vi "Tenney Calculate Setpoint Change.vi"(0 "Average":dbl, 1 "Adjustment Amount":dbl, 5 "Target Upper limit":dbl, 7 "Target Lower limit":dbl, 11 "error in (no error)":errorcluster, 12 "Chamber Upper limit":dbl, 13 "Chamber Lower limit":dbl, 14 "Chamber Setpoint":dbl) -> (4 "new_setpoint":dbl, 15 "error out":errorcluster)   [LabVIEW 2023]
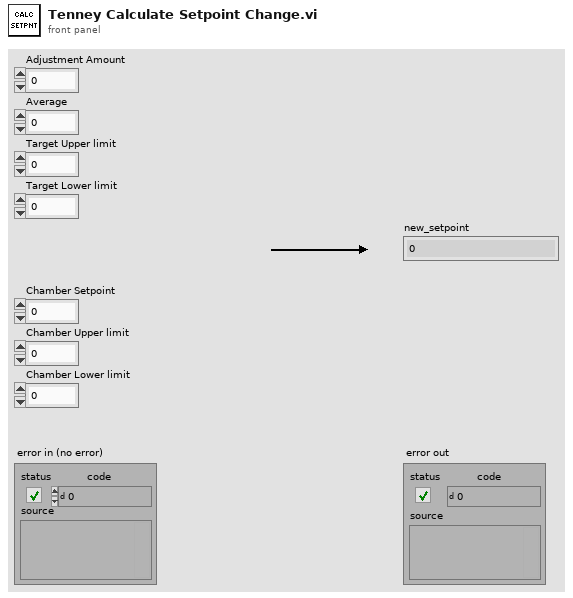
[diagram p1: front panel]
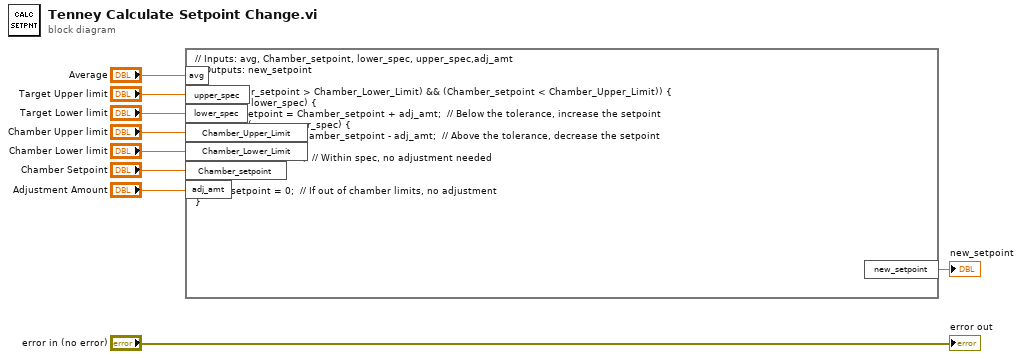
[diagram p0: block diagram]
diagram:
  n1 = formula code="// Inputs: avg, Chamber_setpoint, lower_spec, upper_spec,adj_amt\n// Outputs: new_setpoint\n\nif ((Chamber_setpoint > Chamber_Lower_Limit) && (Chamber_setpoint < Chamber_Upper_Limit)) {\n    if (avg < lower_spec) {\n        new_setpoint = Chamber_setpoint + adj_amt;  // Below the tolerance, increase the setpoint\n    } else if (avg > upper_spec) {\n        new_setpoint = Chamber_setpoint - adj_amt;  // Above the tolerance, decrease the setpoint\n    } else {\n        new_setpoint = 0;  // Within spec, no adjustment needed\n    }\n} else {\n    new_setpoint = 0;  // If out of chamber limits, no adjustment\n}"("avg"="Average", "lower_spec"="Target Lower limit", "upper_spec"="Target Upper limit", "Chamber_setpoint"="Chamber Setpoint", "Chamber_Upper_Limit"="Chamber Upper limit", "Chamber_Lower_Limit"="Chamber Lower limit", "adj_amt"="Adjustment Amount") -> ("new_setpoint"=→"new_setpoint":dbl)
  "error out" <- "error in (no error)"
